vi "Test LRS RT.vi"() -> ()   [LabVIEW 2014]
uses:
  <vilib>/FPGAPlugInAG/sbRIO-9606/niLvFpga_Open_sbRIO-9606.vi
  <vilib>/rvi/interface/common/dynamic/niFpgaDynamicAddResources.vi
  <vilib>/rvi/interface/common/niFpgaWaitOnOcc.vi
  <vilib>/Utility/error.llb/Error Cluster From Error Code.vi
  <vilib>/Analysis/1siggen.llb/Ramp Pattern by Delta.vi
  <vilib>/rvi/errors/niLvFpgaAdjustHostInterfaceError.vi
  <vilib>/FPGAPlugInAG/Dynamic/niLvFpga_Close_Dynamic.vi
  <vilib>/rvi/interface/nirviOpenFPGA/nirviOpenFPGA.xnode
  LRS/FPGA Bitfiles/LRS_FPGA.lvbitx
  <vilib>/rvi/interface/nirviMethod/nirviMethod.xnode
  <vilib>/rvi/interface/nirviReadWriteControl/nirviReadWriteControl.xnode
  <vilib>/rvi/interface/nirviCloseFPGA/nirviCloseFPGA.xnode
  <vilib>/FPGAPlugInAG/Dynamic/niLvFpga_ConfigureFifo_Dynamic.vi
  <vilib>/rvi/errors/niLvFpgaMergeErrorWithErrorCode.vi
  <vilib>/FPGAPlugInAG/Dynamic/niLvFpga_StartFifo_Dynamic.vi
  Reusable/General/Math/Fit Exponential Class/Fit Exponential.lvclass
  <vilib>/FPGAPlugInAG/Dynamic/niLvFpga_WriteFifo_Dynamic.vi
  <vilib>/Analysis/NI_AALBase.lvlib
  NiFpgaLv.dll
  <vilib>/rvi/interface/Simulation/niFpgaSimulationCallBeginRW.vi
panel:
  out "RT":T1 {"Stt" format="%#.2f"}
  in  "end":dbl=499.0 format="%#_13g"
  out "ExecTime":u32
  out "FPGA":T2
  in  "Stop":bool
  in  "Start Calc":bool
  out "Waveform Graph":i16[](graph)
  in  "B":dbl
  in  "A":dbl
  in  "tau":dbl
  in  "Load?":bool
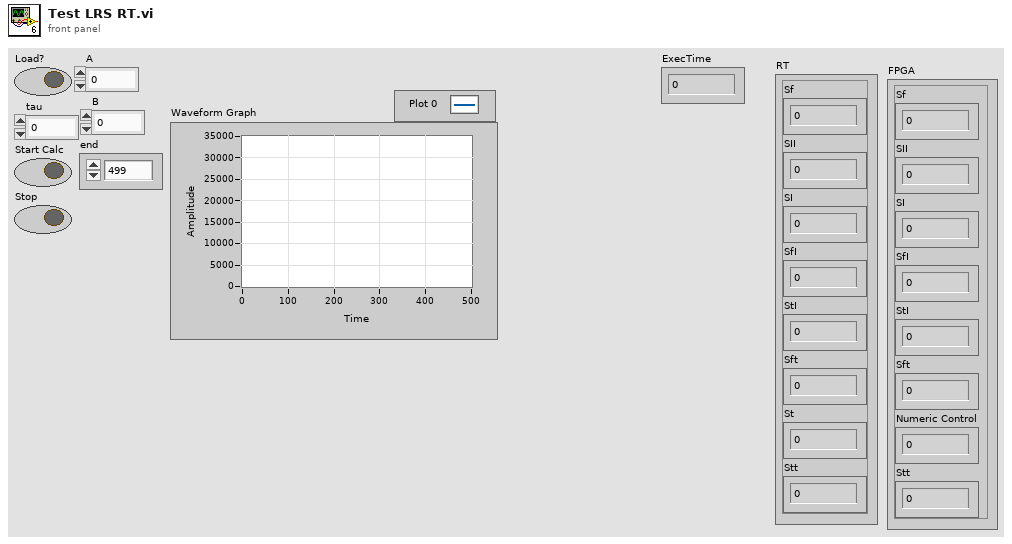
[diagram p1: front panel]
types:
  T1 = cluster{"Sf":i64, "SII":i64, "SI":i64, "SfI":i64, "StI":i64, "Sft":i16, "St":dbl, "Stt":dbl}
  T2 = cluster{"Sf":i32, "SII":i64, "SI":i64, "SfI":i64, "StI":i64, "Sft":i64, "Numeric Control":i32, "Stt":i64}
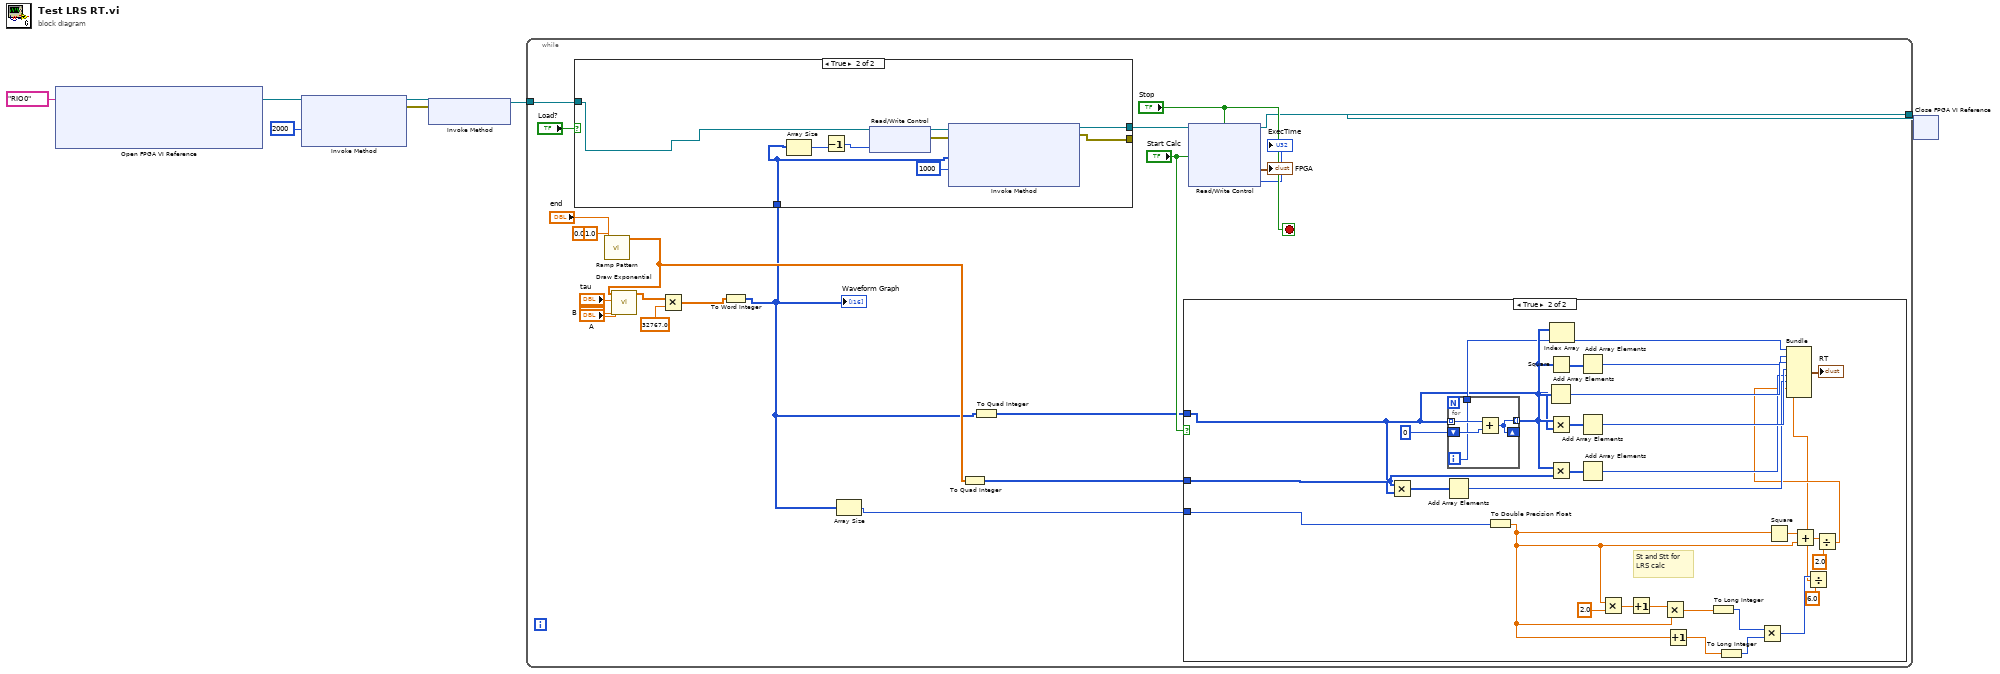
[diagram p0: block diagram]
diagram:
  n1 = xnode "Open FPGA VI Reference"("resource name"=tag "RIO0") -> ("FPGA VI Reference Out"=w6:refnum<k20>)  [unwired: 1 in, 1 out]
  n2 = xnode "Invoke Method"("FPGA VI Reference In"=w6, "Requested Depth"=u32 2000) -> ("FPGA VI Reference Out"=w4:refnum<k20>, "error out"=w3:errorcluster)  [unwired: 1 in, 1 out]
  n3 = xnode "Invoke Method"("FPGA VI Reference In"=w4, "error in"=w3) -> ("FPGA VI Reference Out"=w2:refnum<k20>)  [unwired: 1 out]
  n4 = while {
    tunnel: w2 -> [w28]
    tunnel: [w25] -> w1
    stop <- "Stop" stop-if-true
    n5 = call-poly <vilib>:"Ramp Pattern.vi"("start"=0.0, "end"="end", "delta"=1.0) -> ("Ramp Pattern"=w11:dbl[])  [unwired: 6 in, 2 out]
    n6 = call "Draw Exponential.vi"("B"="B", "A"="A", "tau"="tau", "time"=w11) -> ("ExponentialOut"=w17:dbl[])  [unwired: 7 in]
    n7 = Multiply(x=w17, y=32767.0) -> (x*y=w14:dbl[])
    n8 = To Word Integer(number=w14) -> (16bit integer=w9:i16[])
    "Waveform Graph" <- w9
    n9 = case shown="True" "Load?" {
      tunnel: w28 -> [w66 w70]
      tunnel: [w66 w72] -> w27
      tunnel: [_ w71] -> _
      tunnel: w9 -> [_ w69]
      frame False {
      }
      frame True {
        n10 = Array Size(array=w69) -> (size(s)=w68:i32)
        n11 = Decrement(x=w68) -> (x-1=w67:i32)
        n12 = xnode "Read/Write Control"("FPGA VI Reference In"=w70, "Num2Proc"=w67) -> ("FPGA VI Reference Out"=w75:refnum<k20>, "error out"=w74:errorcluster)  [unwired: 1 in]
        n13 = xnode "Invoke Method"("FPGA VI Reference In"=w75, "error in"=w74, "Data"=w69, "Timeout (ms)"=1000) -> ("FPGA VI Reference Out"=w72:refnum<k20>, "error out"=w71:errorcluster)  [unwired: 1 out]
      }
    }
    n14 = Array Size(array=w9) -> (size(s)=w12:i32)
    n15 = To Quad Integer(1:w11) -> (0:w10:i64[])
    n16 = To Quad Integer(1:w9) -> (0:w8:i64[])
    n17 = case shown="True" "Start Calc" {
      tunnel: w12 -> [_ w35]
      tunnel: w10 -> [_ w57]
      tunnel: w8 -> [_ w30]
      frame False {
      }
      frame True {
        # "St and Stt for LRS calc"
        n18 = Multiply(x=w57, y=w30) -> (x*y=w50:i64[])
        n19 = Add Array Elements ("SfI")(numeric array=w50) -> (sum=w58:i64)
        n20 = for {
          tunnel: w30 -> [w65] mode=indexing
          tunnel: [w63] -> w52 mode=indexing
          shift-right: [w63] -> _
          shift-left: i64 0 -> [w64]
          tunnel: [w62] -> w31
          i -> [w62]
          n21 = Add(x=w65, y=w64) -> (x+y=w63:i64)
        }
        n22 = To Double Precision Float(number=w35) -> (double precision float=w40:dbl)
        n23 = Square(x=w52) -> (x^2=w49:i64[])
        n24 = Add Array Elements ("SII")(numeric array=w52) -> (sum=w61:i64)
        n25 = Multiply(x=w52, y=w30) -> (x*y=w53:i64[])
        n26 = Multiply(x=w52, y=w57) -> (x*y=w51:i64[])
        n27 = Index Array(array=w52, index=w31) -> (element=w56:i64)
        n28 = Add Array Elements ("SII")(numeric array=w49) -> (sum=w55:i64)
        n29 = Add Array Elements ("SfI")(numeric array=w53) -> (sum=w60:i64)
        n30 = Add Array Elements ("SfI")(numeric array=w51) -> (sum=w59:i64)
        n31 = Multiply(x=w40, y=2.0) -> (x*y=w43:dbl)
        n32 = Increment(x=w43) -> (x+1=w42:dbl)
        n33 = Multiply(x=w42, y=w40) -> (x*y=w39:dbl)
        n34 = Increment(x=w40) -> (x+1=w38:dbl)
        n35 = To Long Integer(number=w39) -> (32bit integer=w36:i32)
        n36 = To Long Integer(number=w38) -> (32bit integer=w37:i32)
        n37 = Multiply(x=w36, y=w37) -> (x*y=w41:i32)
        n38 = Square(x=w40) -> (x^2=w45:dbl)
        n39 = Add(x=w45, y=w40) -> (x+y=w46:dbl)
        n40 = Divide(x=w41, y=6.0) -> (x/y=w33:dbl)
        n41 = Divide(x=w46, y=2.0) -> (x/y=w34:dbl)
        n42 = Bundle(w56, w55, w61, w60, w59, w58, w34, w33) -> (→"RT":cluster{i64, i64, i64, i64, i64, i64, dbl, dbl})  [unwired: 1 in]
      }
    }
    n43 = xnode "Read/Write Control"("FPGA VI Reference In"=w27, "Stop"="Stop", "Start Calc"="Start Calc") -> ("FPGA VI Reference Out"=w25:refnum<k20>, "OutputParms"=→"FPGA":T2, "ExecTime"=→"ExecTime":u32)  [unwired: 1 in, 1 out]
  }
  n44 = xnode "Close FPGA VI Reference"("FPGA VI Reference In"=w1) -> ()  [unwired: 1 in, 1 out]
